vi "unit test.vi"() -> ()   [LabVIEW 2018]
uses:
  Desktop/builds/Control Box.lvlibp/Custom Controls/Channel Status.ctl
  Desktop/builds/Control Box.lvlibp/Control Box.lvclass
  Desktop/builds/Control Box.lvlibp
panel:
  out "Control Board":T1
  out "Channel Status":T1[](array[typedef])
  out "error out":errorcluster
  in  "stop":bool
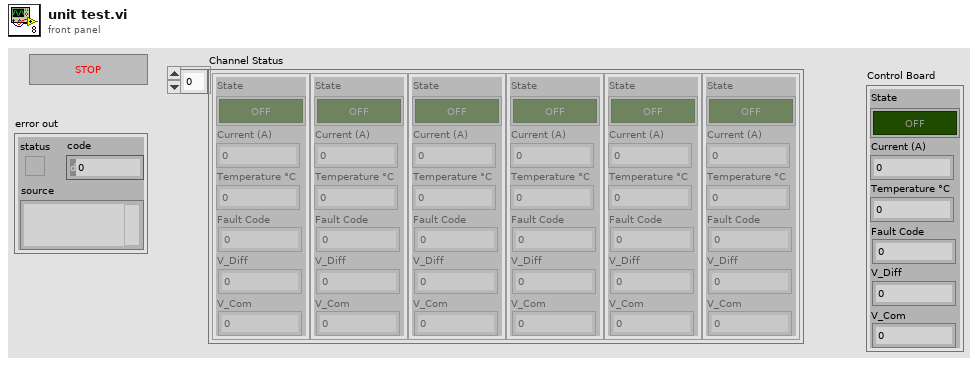
[diagram p1: front panel]
types:
  T1 = typedef "Control Box.lvlibp/Channel Status.ctl" = cluster{"State":bool, "Current (A)":dbl, "Temperature °C":dbl, "Fault Code":u8, "V_Diff":dbl, "V_Com":dbl}
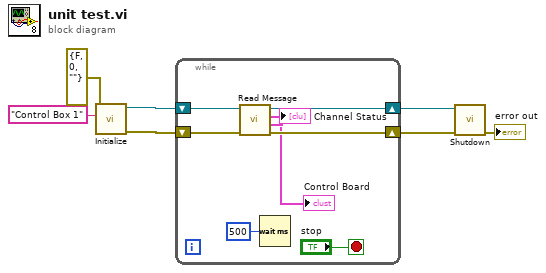
[diagram p0: block diagram]
diagram:
  n1 = call "Initialize.vi"("error in"=errorcluster {"status"=FALSE, "code"=0, "source"=""}, "Device"="Control Box 1") -> ("error out"=w6:errorcluster, "Control Box out"=w7:refnum<class "Control Box.lvclass">)  [unwired: 8 in]
  n2 = while {
    shift-right: [w13] -> w5
    shift-left: w7 -> [w15]
    shift-right: [w12] -> w4
    shift-left: w6 -> [w14]
    stop <- "stop" stop-if-true
    n3 = call "Read Message.vi"("error in (no error)"=w14, "Control Box in"=w15) -> ("error out"=w12:errorcluster, "Remaining Channels"=→"Channel Status":T1[], "Control Board"=→"Control Board":T1, "Control Box out"=w13:refnum<class "Control Box.lvclass">)  [unwired: 6 in]
    n4 = Wait (ms)(milliseconds to wait=u32 500) -> ()  [unwired: 1 out]
  }
  n5 = call "Shutdown.vi"("error in"=w4, "Control Box in"=w5) -> ("error out"=→"error out":errorcluster)  [unwired: 8 in, 1 out]
